vi "trash_Load Payload.vi"(8 "error in (no error)":errorcluster, 10 "Configuration Payload":variant, 11 "CoreOOB_Rx in":refnum<class "ChanMngOOB_Rx.lvclass">) -> (0 "error out":errorcluster, 3 "CoreOOB_Rx out":refnum<class "ChanMngOOB_Rx.lvclass">)   [LabVIEW 2021]
uses:
  ChanMngOOB_Rx.lvclass/ChanMngOOB_Rx.ctl
  Typedef/Template Payload.ctl
  ChanMngOOB_Rx.lvclass
  <vilib>/CIF Foundation/CIF Out of Band Commands/CIFOutOfBand.lvclass
  C:/Program Files/National Instruments/LabVIEW 2021/vi.lib/CIF Foundation/CIF Out of Band Commands/CIFOutOfBand.lvclass
  Typedef/Channel Connection Data.ctl
  Typedef/Channel Fault Data.ctl
  <vilib>/CIF Foundation/CIF Channels Core/ChannelCommon/typedef/New FIFO Instance Configuration.ctl
  <vilib>/CIF Foundation/CIF Channels Core/ChannelCommon/ChannelCommon.lvlib
  Typedef/New FIFO Publisher.ctl
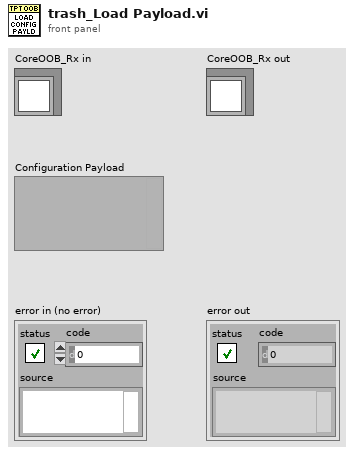
[diagram p1: front panel]
types:
  T1 = typedef "ChanMngOOB_Rx.lvclass/Template Payload.ctl" = cluster{"Connections":T2[], "Forces":T3[], "New FIFO Pub":T4}
  T2 = typedef "ChanMngOOB_Rx.lvclass/Channel Connection Data.ctl" = cluster{"Publisher Name":string, "Subscriber Name":string, "Connection Data":u8[]}
  T3 = typedef "ChanMngOOB_Rx.lvclass/Channel Fault Data.ctl" = cluster{"Channel Name":string, "Force Data":u8[], "Force Active":bool}
  T4 = typedef "ChanMngOOB_Rx.lvclass/New FIFO Publisher.ctl" = cluster{"Publisher Name":string, "New FIFO Instance Config":T5}
  T5 = typedef "ChannelCommon.lvlib/New FIFO Instance Configuration.ctl" = cluster{"Primary":bool, "Backpressure":bool, "Message/FIFO Override":u32}
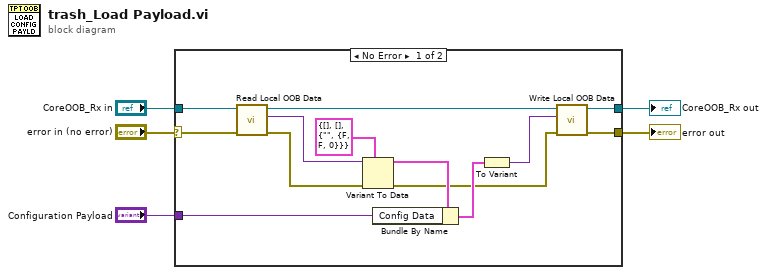
[diagram p0: block diagram]
diagram:
  n1 = case shown="No Error" "error in (no error)" {
    selector: "error in (no error)" -> [w10 w20]
    tunnel: [w18 w20] -> w5
    tunnel: [w17 w19] -> w4
    tunnel: "CoreOOB_Rx in" -> [w13 w19]
    tunnel: "Configuration Payload" -> [w16 _]
    frame No Error {
      n2 = call <vilib>:"Read Local OOB Data.vi"("error in"=w10, "OOB in"=w13) -> ("error out"=w7:errorcluster, "Local OOB Data"=w11:variant, "OOB out"=w12:refnum<class "ChanMngOOB_Rx.lvclass">)  [unwired: 7 in]
      n3 = Variant To Data(error in=w7, type=T1 {"Connections"=[], "Forces"=[], "New FIFO Pub"={"Publisher Name"="", "New FIFO Instance Config"={"Primary"=FALSE, "Backpressure"=FALSE, "Message/FIFO Override"=0}}} ("Template Payload"), Variant=w11) -> (data=w8:T1, error out=w6:errorcluster)
      n4 = Bundle By Name(cluster=w8, "Config Data"=w16) -> (w15:T1)
      n5 = To Variant(anything=w15) -> (Variant=w14:variant)
      n6 = call <vilib>:"Write Local OOB Data.vi"("error in"=w6, "Local OOB Data"=w14, "OOB in"=w12) -> ("error out"=w18:errorcluster, "OOB out"=w17:refnum<class "ChanMngOOB_Rx.lvclass">)  [unwired: 7 in]
    }
    frame Error {
    }
  }
  "error out" <- w5
  "CoreOOB_Rx out" <- w4
